vi "Get Child.vi"(8 "error in (no error)":errorcluster, 11 "NodeRef In":refnum<data-value>) -> (0 "error out":errorcluster, 2 "Child":refnum<data-value>, 3 "NodeRef":refnum<data-value>)   [LabVIEW 2020, in "PicoG-ParserLexer.lvlib" / "Node.lvclass"]
uses:
  Node.lvclass
  Node.lvclass/Node.ctl
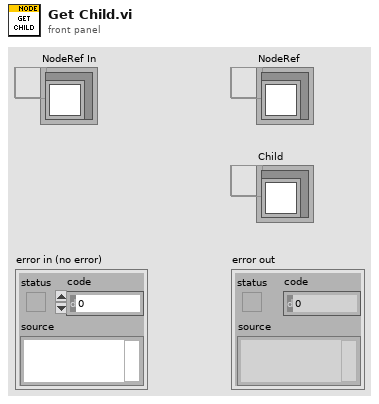
[diagram p1: front panel]
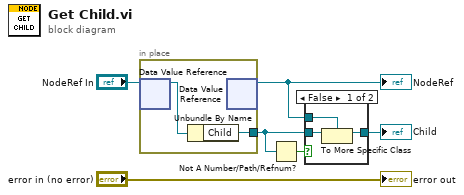
[diagram p0: block diagram]
diagram:
  n1 = in-place {
    in-place-border: [w7] -> w3
    n2 = in-place-dvr #1("NodeRef In") -> (w8:refnum<class "Node.lvclass">)  [unwired: 1 out]
    n3 = Unbundle By Name(w8) -> ("Child"=w7:refnum<data-value>)
    n4 = in-place-dvr #1() -> (w2:refnum<data-value>)  [unwired: 1 in, 1 out]
  }
  "NodeRef" <- w2
  n5 = Not A Number/Path/Refnum?(number/path/refnum=w3) -> (NaN/Path/Refnum?=w4:bool)
  n6 = case shown="False" w4 {
    tunnel: w3 -> [w11 _]
    tunnel: w2 -> [w10 _]
    tunnel: [w9 _] -> w1
    frame False {
      n7 = To More Specific Class(target class=w10, reference=w11) -> (specific class reference=w9:refnum<data-value>)  [unwired: 1 in, 1 out]
    }
    frame True {
    }
  }
  "Child" <- w1
  "error out" <- "error in (no error)"
